vi "adjuststoplength.vi"() -> ()   [LabVIEW 2013]
uses:
  Reinitializecontrol.ctl
panel:
  out "Motor Output":dbl
  in  "Boolean":bool
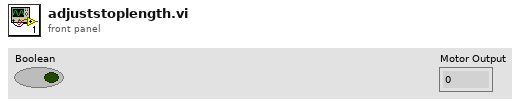
[diagram p1: front panel]
types:
  T1 = typedef "Reinitializecontrol.ctl" = enum16{"Nonzero", "FollowingZero", "FirstZero"}
  T2 = typedef "WPI_MotorControlDeviceRef.ctl" = cluster{"DeviceStatus":errorcluster, "Type":enum16{"PWM", "CAN"}, "PWM":cluster{"Digital Module":T3, "PWM Channel":T4, "DeadBand":T5}, "CAN":cluster{"Device Number":u8, "Control Mode":T6, "Semaphore":T7, "Max Vout":dbl}, "Invert":bool, "TransformRef":T8, "InvTransformRef":T8}
  T3 = typedef "FPGA_TypedefDigitalModule.ctl" = enum16{"Digital Module 1", "Digital Module 2"}
  T4 = typedef "FPGA_DIOPWMChannel.ctl" = enum8{"PWM 1", "PWM 2", "PWM 3", "PWM 4", "PWM 5", "PWM 6", "PWM 7", "PWM 8", "PWM 9", "PWM 10", "Invalid"}
  T5 = typedef "WPI_PWMDeadband.ctl" = cluster{"Name":string, "maxPositivePwm":i32, "minPositivePwm":i32, "centerPwm":i32, "maxNegativePwm":i32, "minNegativePwm":i32, "angularRange":u16}
  T6 = typedef "WPI_CANJaguar_ControlMode.ctl" = enum8{"Percent VBus", "Current", "Speed", "Position", "Voltage"}
  T7 = typedef "Semaphore RefNum" = refnum<k1>
  T8 = typedef "WPI_PWMTransform_ConPane.ctl" = refnum<vi>
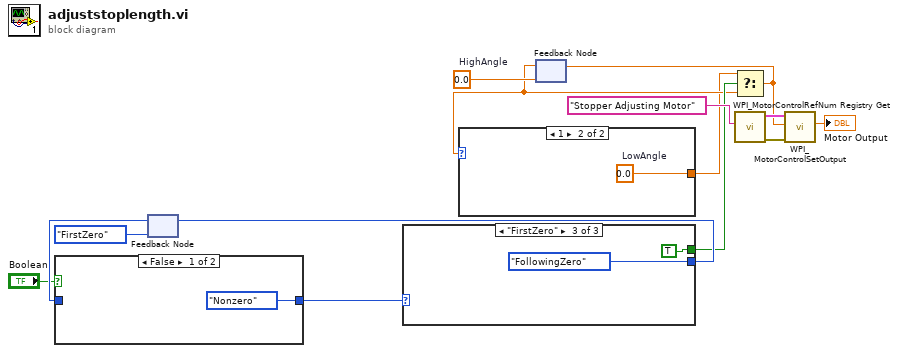
[diagram p0: block diagram]
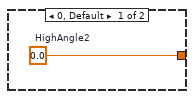
[diagram p2: hidden frame]
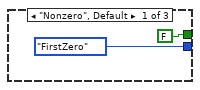
[diagram p4: hidden frame]
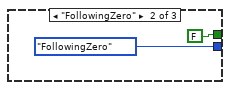
[diagram p5: hidden frame]
diagram:
  w6 = 0.0  # HighAngle
  n1 = feedback #1(Reinitializecontrol."FirstZero") -> (w9:T1)
  n2 = case shown="False" "Boolean" {
    tunnel: [Reinitializecontrol."Nonzero" w16] -> w10
    tunnel: w9 -> [_ w16]
    frame False {
    }
    frame True {
    }
  }
  n3 = case shown="\"FirstZero\"" w10 {
    tunnel: [Reinitializecontrol."FirstZero" Reinitializecontrol."FollowingZero" Reinitializecontrol."FollowingZero"] -> w8
    tunnel: [FALSE ("reinitialize? (F)") FALSE ("reinitialize? (F)") TRUE ("reinitialize? (F)")] -> w7
    frame "Nonzero", Default {
    }
    frame "FollowingZero" {
    }
    frame "FirstZero" {
    }
  }
  n4 = feedback-in #1(w8) -> ()
  n5 = feedback #2(w6) -> (w5:dbl)
  n6 = case shown="1" w5 {
    tunnel: [w23 w24] -> w4
    frame 0, Default {
      w23 = 0.0  # HighAngle2
    }
    frame 1 {
      w24 = 0.0  # LowAngle
    }
  }
  n7 = Select(t=w4, s=w7, f=w5) -> (s? t:f=w3:dbl)
  n8 = feedback-in #2(w3) -> ()
  n9 = call <vilib>:"WPI_MotorControlRefNum Registry Get.vi"("refnum name"="Stopper Adjusting Motor") -> ("error out"=w13:errorcluster, "MotorControlDevRef"=w12:T2)  [unwired: 9 in]
  n10 = call <vilib>:"WPI_MotorControlSetOutput.vi"("error in (no error)"=w13, "Output"=w3, "MotorControlDevRef"=w12) -> ("Motor Output"=→"Motor Output":dbl)  [unwired: 6 in, 2 out]
